vi "Current Channels Array.vi"(8 "error in":errorcluster, 11 "Channel 1":string) -> (0 "error out":errorcluster, 1 "Current Channel?":bool, 2 "Channel 2":string, 3 "Channel 1":string)   [LabVIEW 2021, in "DMM_Scan PXI RLY Driver 32V-16C.lvlib"]
doc: "Checks if the channel is a current channel (channels 32 to 47) and provides chX+16 and comX+16 names for individual current shunt relay paths (48 to 63 will be reserved).\n\nReturns if Channel 1 is part of a current channel mapping."
uses:
  DMM_Scan PXI RLY Driver 32V-16C.lvlib
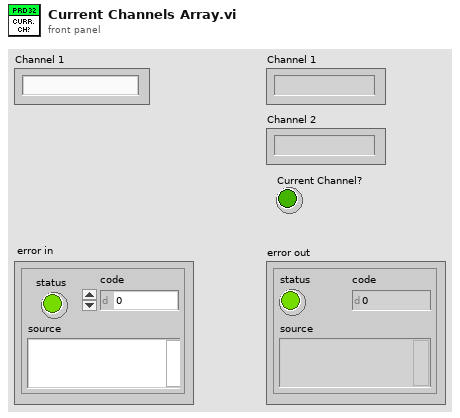
[diagram p1: front panel]
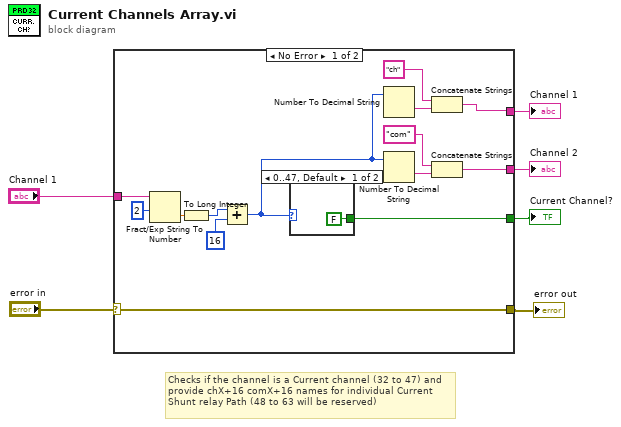
[diagram p0: block diagram]
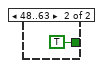
[diagram p2: hidden frame]
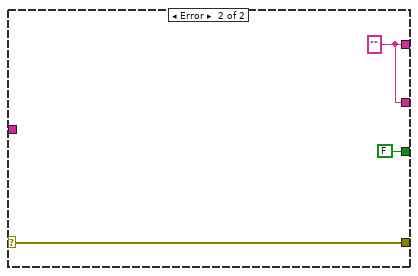
[diagram p3: hidden frame]
diagram:
  # "Checks if the channel is a Current channel (32 to 47) and provide chX+16 comX+16 names for individual Current Shunt relay Path (48 to 63 will be reserved)"
  n1 = case shown="No Error" "error in" {
    selector: "error in" -> [w18 w25]
    tunnel: "Channel 1" -> [w12 _]
    tunnel: [w18 w25] -> w1
    tunnel: [w17 FALSE] -> w5
    tunnel: [w13 w23] -> w4
    tunnel: [w7 w23] -> w3
    frame No Error {
      n2 = Fract/Exp String To Number(string=w12, offset=2 ("offset (0)")) -> (number=w19:dbl)  [unwired: 2 in, 1 out]
      n3 = To Long Integer(number=w19) -> (32bit integer=w14:i32)
      n4 = Add(x=w14, y=16 ("offset (0)")) -> (x+y=w8:i32)
      n5 = case shown="0..47, Default" w8 {
        tunnel: [FALSE TRUE] -> w17
        frame 0..47, Default {
        }
        frame 48..63 {
        }
      }
      n6 = Number To Decimal String(number=w8) -> (decimal integer string=w9:string)  [unwired: 1 in]
      n7 = Number To Decimal String(number=w8) -> (decimal integer string=w16:string)  [unwired: 1 in]
      n8 = Concatenate Strings("ch", w9) -> (w7:string)
      n9 = Concatenate Strings("com", w16) -> (w13:string)
    }
    frame Error {
      w23 = ""
    }
  }
  "Current Channel?" <- w5
  "Channel 2" <- w4
  "Channel 1" <- w3
  "error out" <- w1
